vi "Clear_Old_Files.vi"(10 "Bash Script Folder Name":string="Wavedump_Bash_Script_Test_", 11 "Channel":string[](array[string])) -> ()   [LabVIEW 2018]
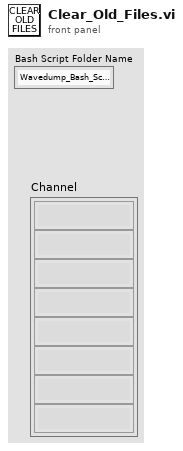
[diagram p1: front panel]
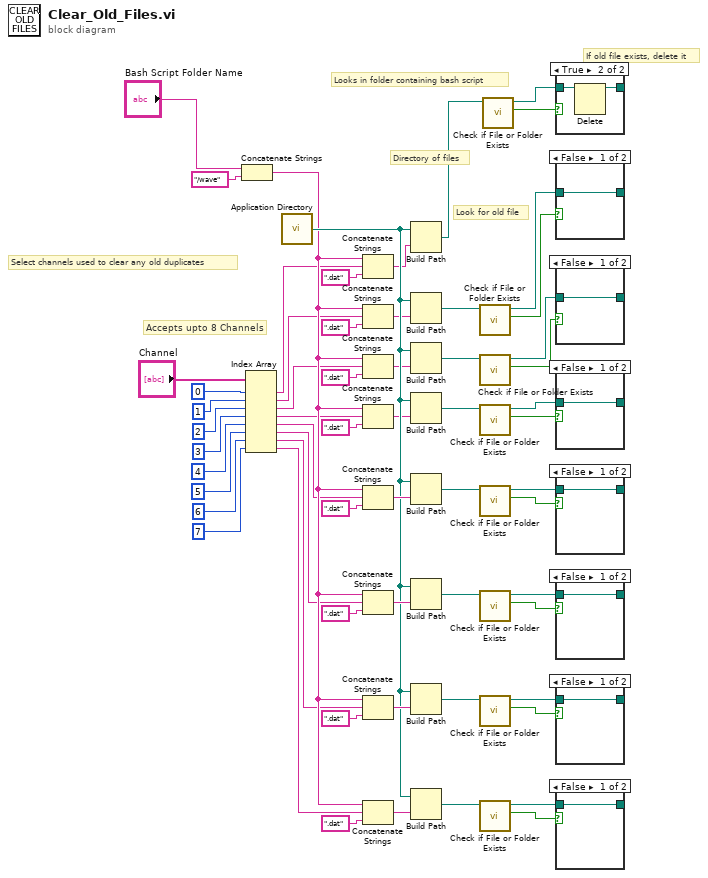
[diagram p0: block diagram]
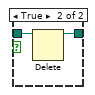
[diagram p2: hidden frame]
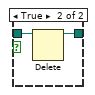
[diagram p3: hidden frame]
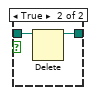
[diagram p4: hidden frame]
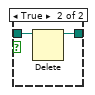
[diagram p5: hidden frame]
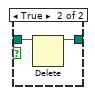
[diagram p6: hidden frame]
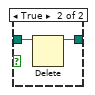
[diagram p7: hidden frame]
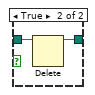
[diagram p8: hidden frame]
diagram:
  # "Accepts upto 8 Channels"
  # "Select channels used to clear any old duplicates"
  # "Looks in folder containing bash script"
  # "Directory of files"
  # "Look for old file"
  # "If old file exists, delete it"
  n1 = Concatenate Strings("Bash Script Folder Name", "/wave" ("string")) -> (w46:string)
  n2 = Index Array(array="Channel", index #1=0 ("index"), index #2=1 ("index"), index #3=2 ("index"), index #4=3 ("index"), index #5=4 ("index"), index #6=5 ("index"), index #7=6 ("index"), index #8=7 ("index")) -> (element #1=w31:string, element #2=w39:string, element #3=w40:string, element #4=w41:string, element #5=w42:string, element #6=w43:string, element #7=w44:string, element #8=w45:string)
  n3 = call <vilib>:"Application Directory.vi"() -> ("Application Directory"=w51:path)
  n4 = Concatenate Strings(w46, w31, ".dat" ("string")) -> (w20:string)
  n5 = Concatenate Strings(w46, w39, ".dat" ("string")) -> (w48:string)
  n6 = Concatenate Strings(w46, w40, ".dat" ("string")) -> (w47:string)
  n7 = Concatenate Strings(w46, w41, ".dat" ("string")) -> (w49:string)
  n8 = Concatenate Strings(w46, w42, ".dat" ("string")) -> (w52:string)
  n9 = Concatenate Strings(w46, w43, ".dat" ("string")) -> (w53:string)
  n10 = Concatenate Strings(w46, w44, ".dat" ("string")) -> (w54:string)
  n11 = Concatenate Strings(w46, w45, ".dat" ("string")) -> (w55:string)
  n12 = Build Path(base path=w51, name or relative path=w20) -> (appended path=w32:path)
  n13 = Build Path(base path=w51, name or relative path=w48) -> (appended path=w50:path)
  n14 = Build Path(base path=w51, name or relative path=w47) -> (appended path=w56:path)
  n15 = Build Path(base path=w51, name or relative path=w49) -> (appended path=w57:path)
  n16 = Build Path(base path=w51, name or relative path=w52) -> (appended path=w58:path)
  n17 = Build Path(base path=w51, name or relative path=w53) -> (appended path=w61:path)
  n18 = Build Path(base path=w51, name or relative path=w54) -> (appended path=w59:path)
  n19 = Build Path(base path=w51, name or relative path=w55) -> (appended path=w60:path)
  n20 = call <vilib>:"Check if File or Folder Exists.vi"("path"=w50) -> ("file or folder exists?"=w5:bool, "dup path"=w4:path)  [unwired: 8 in, 1 out]
  n21 = call <vilib>:"Check if File or Folder Exists.vi"("path"=w56) -> ("file or folder exists?"=w7:bool, "dup path"=w6:path)  [unwired: 8 in, 1 out]
  n22 = call <vilib>:"Check if File or Folder Exists.vi"("path"=w57) -> ("file or folder exists?"=w9:bool, "dup path"=w8:path)  [unwired: 8 in, 1 out]
  n23 = call <vilib>:"Check if File or Folder Exists.vi"("path"=w58) -> ("file or folder exists?"=w11:bool, "dup path"=w10:path)  [unwired: 8 in, 1 out]
  n24 = call <vilib>:"Check if File or Folder Exists.vi"("path"=w61) -> ("file or folder exists?"=w13:bool, "dup path"=w12:path)  [unwired: 8 in, 1 out]
  n25 = call <vilib>:"Check if File or Folder Exists.vi"("path"=w59) -> ("file or folder exists?"=w15:bool, "dup path"=w14:path)  [unwired: 8 in, 1 out]
  n26 = call <vilib>:"Check if File or Folder Exists.vi"("path"=w60) -> ("file or folder exists?"=w17:bool, "dup path"=w16:path)  [unwired: 8 in, 1 out]
  n27 = call <vilib>:"Check if File or Folder Exists.vi"("path"=w32) -> ("file or folder exists?"=w3:bool, "dup path"=w2:path)  [unwired: 8 in, 1 out]
  n28 = case shown="True" w3 {
    tunnel: w2 -> [w62 w64]
    tunnel: [w62 w63] -> _
    frame False {
    }
    frame True {
      n29 = Delete(path (use dialog)=w64) -> (deleted path=w63:path)  [unwired: 4 in, 2 out]
    }
  }
  n30 = case shown="False" w5 {
    tunnel: w4 -> [w65 w67]
    tunnel: [w65 w66] -> _
    frame False {
    }
    frame True {
      n31 = Delete(path (use dialog)=w67) -> (deleted path=w66:path)  [unwired: 4 in, 2 out]
    }
  }
  n32 = case shown="False" w7 {
    tunnel: w6 -> [w68 w70]
    tunnel: [w68 w69] -> _
    frame False {
    }
    frame True {
      n33 = Delete(path (use dialog)=w70) -> (deleted path=w69:path)  [unwired: 4 in, 2 out]
    }
  }
  n34 = case shown="False" w9 {
    tunnel: w8 -> [w71 w73]
    tunnel: [w71 w72] -> _
    frame False {
    }
    frame True {
      n35 = Delete(path (use dialog)=w73) -> (deleted path=w72:path)  [unwired: 4 in, 2 out]
    }
  }
  n36 = case shown="False" w11 {
    tunnel: w10 -> [w74 w76]
    tunnel: [w74 w75] -> _
    frame False {
    }
    frame True {
      n37 = Delete(path (use dialog)=w76) -> (deleted path=w75:path)  [unwired: 4 in, 2 out]
    }
  }
  n38 = case shown="False" w13 {
    tunnel: w12 -> [w77 w79]
    tunnel: [w77 w78] -> _
    frame False {
    }
    frame True {
      n39 = Delete(path (use dialog)=w79) -> (deleted path=w78:path)  [unwired: 4 in, 2 out]
    }
  }
  n40 = case shown="False" w15 {
    tunnel: w14 -> [w80 w82]
    tunnel: [w80 w81] -> _
    frame False {
    }
    frame True {
      n41 = Delete(path (use dialog)=w82) -> (deleted path=w81:path)  [unwired: 4 in, 2 out]
    }
  }
  n42 = case shown="False" w17 {
    tunnel: w16 -> [w83 w85]
    tunnel: [w83 w84] -> _
    frame False {
    }
    frame True {
      n43 = Delete(path (use dialog)=w85) -> (deleted path=w84:path)  [unwired: 4 in, 2 out]
    }
  }
